vi "Read Measurement Data (Digital NChan).vi"(0 "VISA resource name":refnum<visa-resource-name>, 5 "Start Channel (1)":string="0001", 7 "End Channel (1)":string="0001", 9 "Data Format (0 : Binary)":i32(ring) items=["Binary", "ASCII"], 11 "error in (no error)":errorcluster) -> (2 "Date Time":timestamp=timestamp(3345116400 s since 1904-01-01) format="%<%H:%M:%S%3u\n%x>T", 4 "VISA resource name out":refnum<visa-resource-name>, 6 "Channel":string[](array[string]), 8 "Data":u16[](array[numeric]), 10 "Data Status":i32[](array[ring]) items=["Normal", "Differential Input", "Skip", "Over", "Error", "Burnout", "Power Failure"], 13 "Alarm Status":i32[][](array[ring]) items=["No Alarm", "High Limit Alarm (H)", "Low Limit Alarm (L)", "Difference High Limit Alarm (h)", "Difference Low Limit Alarm (l)", "High Limit on Rate-of-change Alarm (R)", "Low Limit on Rate-of-change Alarm (r)", "Delay High Limit Alarm (T)", "Delay Low Limit Alarm (t)"], 15 "error out":errorcluster)   [LabVIEW 2020, in "Yokogawa GX Series.lvlib"]
doc: "This VI reads the digital measurement data by ASCII or Binary."
uses:
  <instrlib>/Yokogawa GX Series/Yokogawa GX Series.lvlib
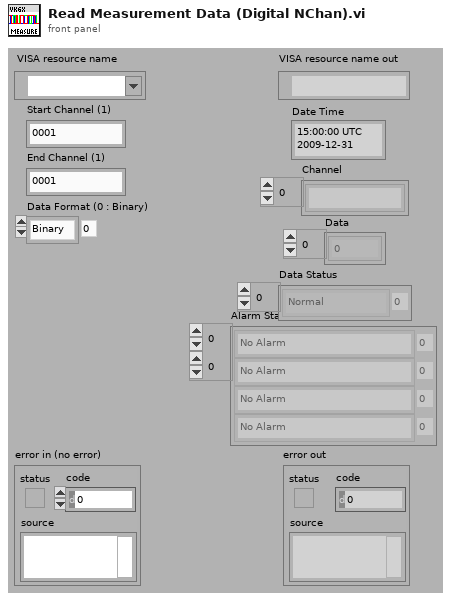
[diagram p1: front panel]
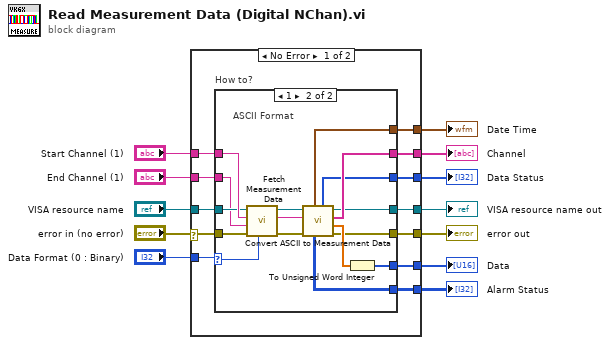
[diagram p0: block diagram]
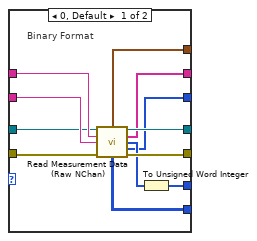
[diagram p2: hidden frame]
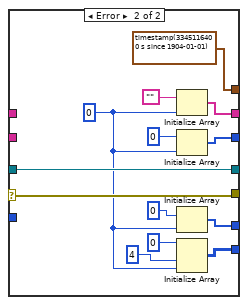
[diagram p3: hidden frame]
diagram:
  n1 = case shown="No Error" "error in (no error)" {
    selector: "error in (no error)" -> [w13 w64]
    tunnel: "VISA resource name" -> [w24 w65]
    tunnel: [w23 w65] -> w11
    tunnel: [w22 w64] -> w10
    tunnel: "Data Format (0 : Binary)" -> [w21 _]
    tunnel: [w20 timestamp(3345116400 s since 1904-01-01)] -> w8
    tunnel: [w19 w62] -> w7
    tunnel: [w18 w57] -> w6
    tunnel: [w17 w55] -> w5
    tunnel: [w16 w61] -> w4
    tunnel: "End Channel (1)" -> [w15 _]
    tunnel: "Start Channel (1)" -> [w14 _]
    frame No Error {
      n2 = case "How to?" shown="1" w21 {
        selector: w21 -> [_ w37]
        tunnel: w24 -> [w34 w51]
        tunnel: w13 -> [w33 w50]
        tunnel: [w32 w40] -> w23
        tunnel: [w31 w43] -> w22
        tunnel: w15 -> [w35 w42]
        tunnel: w14 -> [w36 w52]
        tunnel: [w30 w41] -> w20
        tunnel: [w29 w46] -> w19
        tunnel: [w27 w39] -> w18
        tunnel: [w26 w44] -> w16
        tunnel: [w25 w38] -> w17
        frame 0, Default {
          # "Binary Format"
          n3 = call <instrlib>:"Read Measurement Data (Raw NChan).vi"("VISA resource name"=w34, "Start Channel (1)"=w36, "End Channel (1)"=w35, "error in (no error)"=w33) -> ("Date Time"=w30:timestamp, "VISA resource name out"=w32:refnum<visa-resource-name>, "Channel"=w29:string[], "Data"=w28:i32[], "Data Status"=w26:i32[], "Alarm Status"=w25:i32[][], "error out"=w31:errorcluster)  [unwired: 5 out]
          n4 = To Unsigned Word Integer(number=w28) -> (unsigned 16bit integer=w27:u16[])
        }
        frame 1 {
          # "ASCII Format"
          n5 = call <instrlib>:"Fetch Measurement Data.vi"("Data Format (0 : Binary)"=w37, "error in (no error)"=w50, "End Channel (1)"=w42, "Start Channel (1)"=w52, "VISA resource name"=w51) -> ("error out"=w47:errorcluster, "Measurement Data"=w48:string, "VISA resource name out"=w49:refnum<visa-resource-name>)  [unwired: 4 out]
          n6 = call <instrlib>:"Convert ASCII to Measurement Data.vi"("error in (no error)"=w47, "Measurement ASCII Data (\"\")"=w48, "VISA resource name"=w49) -> ("error out"=w43:errorcluster, "Data"=w45:dbl[], "Channel"=w46:string[], "VISA resource name out"=w40:refnum<visa-resource-name>, "Data Status"=w44:i32[], "Alarm Status"=w38:i32[][], "Date Time"=w41:timestamp)  [unwired: 2 out]
          n7 = To Unsigned Word Integer(number=w45) -> (unsigned 16bit integer=w39:u16[])
        }
      }
    }
    frame Error {
      w53 = 0
      n8 = Initialize Array("", w53) -> (w62:string[])
      n9 = Initialize Array(0, w53) -> (w61:i32[])
      n10 = Initialize Array(u16 0, w53) -> (w57:u16[])
      n11 = Initialize Array(0, 4, w53) -> (w55:i32[][])
    }
  }
  "error out" <- w10
  "VISA resource name out" <- w11
  "Channel" <- w7
  "Alarm Status" <- w5
  "Date Time" <- w8
  "Data" <- w6
  "Data Status" <- w4
